vi "V7310.Example.SetJob.vi"() -> ()   [LabVIEW 2016]
panel:
  out "Jobs with error":string[](array[string])
  out "error IO":errorcluster
  out "size":i32
  out "idx":i32
  out "size(s)":i32
  out "Jobs":string[](array[string])
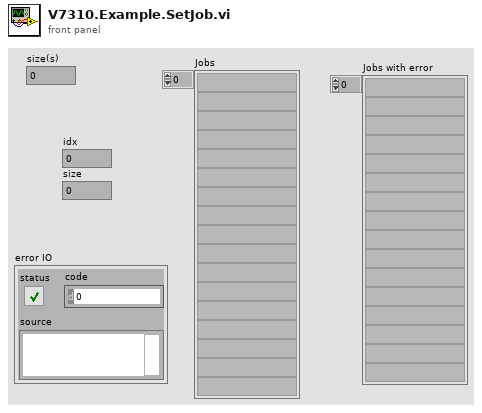
[diagram p1: front panel]
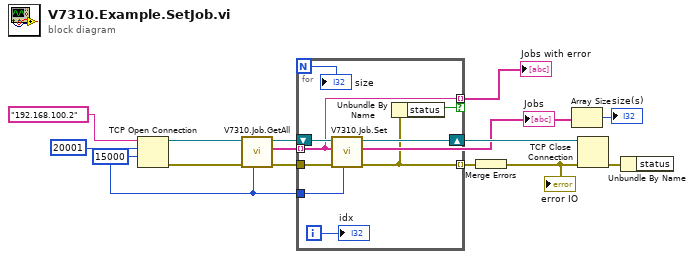
[diagram p0: block diagram]
diagram:
  w7 = 15000 ("timeout ms (60000)")
  n1 = TCP Open Connection(address="192.168.100.2", remote port or service name=u16 20001, timeout ms (60000)=w7) -> (connection ID=w10:refnum<k5>, error out=w9:errorcluster)  [unwired: 2 in]
  n2 = call "V7310.Job.GetAll.vi"("timeout ms (5000)"=w7, "error in"=w9, "Connection in"=w10) -> ("error out"=w4:errorcluster, "Jobs"=w6:string[], "Connection out"=w3:refnum<k5>)  [unwired: 6 in]
  "Jobs" <- w6
  n3 = for {
    N -> [w19]
    tunnel: w6 -> [w17] mode=indexing
    tunnel: w4 -> [w23]
    tunnel: [w16] -> w2 mode=indexing
    shift-right: [w21] -> w12
    shift-left: w3 -> [w22]
    tunnel: w7 -> [w18]
    tunnel: [w17] -> w1 mode=indexing if=w15
    i -> [w20]
    n4 = call "V7310.Job.Set.vi"("timeout ms (5000)"=w18, "error in"=w23, "Job"=w17, "Connection in"=w22) -> ("error out"=w16:errorcluster, "Connection out"=w21:refnum<k5>)  [unwired: 6 in]
    n5 = Unbundle By Name(w16) -> ("status"=w15:bool)
    "idx" <- w20
    "size" <- w19
  }
  "Jobs with error" <- w1
  n6 = Merge Errors(w2) -> (w11:errorcluster)
  "error IO" <- w11
  n7 = Array Size(array=w6) -> (size(s)=→"size(s)":i32)
  n8 = TCP Close Connection(connection ID=w12, error in (no error)=w11) -> (error out=w13:errorcluster)  [unwired: 1 in, 1 out]
  n9 = Unbundle By Name(w13) -> ()  [unwired: 1 out]
